vi "Get homing DSP402.vi"(1 "DSP402 in":refnum<class "DSP402.lvclass">) -> (0 "Done?":bool)   [LabVIEW 2026, in "canopen_.lvlib" / "DSP402.lvclass"]
uses:
  DSP402.lvclass
  DSP402.lvclass/DSP402.ctl
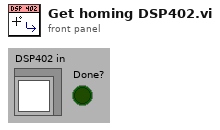
[diagram p1: front panel]
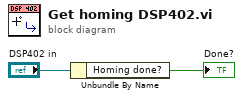
[diagram p0: block diagram]
diagram:
  n1 = Unbundle By Name("DSP402 in") -> ("Homing done?"=→"Done?":bool)
